vi "LabVIEW Version to String.vi"(8 "Error In":errorcluster, 11 "LabVIEW Version":T1) -> (0 "Error Out":errorcluster, 3 "LabVIEW Version":string)   [LabVIEW 2011, in "LVH-Toolbox.lvlib" / "LVH-Common.lvlib"]
uses:
  LVH-Common.lvlib
  Type Defs/LabVIEW Version.ctl
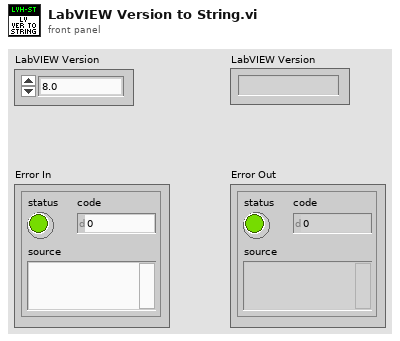
[diagram p1: front panel]
types:
  T1 = typedef "LVH-Toolbox.lvlib/LVH-Common.lvlib/LabVIEW Version.ctl" = enum16{"8.0", "8.2", "8.6", "9.0", "10.0", "11.0", "12.0", "13.0"}
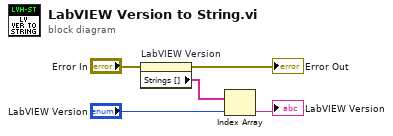
[diagram p0: block diagram]
diagram:
  n1 = property on="LabVIEW Version" class="Enum (strict)"(error in="Error In") -> (error out=→"Error Out":errorcluster, "Strings []"=w3:string[])  [unwired: 1 in, 1 out]
  n2 = Index Array(array=w3, index="LabVIEW Version") -> (element=→"LabVIEW Version":string)
